vi "Add Value.vi"(8 "error in (no error)":errorcluster, 9 "Value":refnum<class>, 10 "Path":string, 11 "PathTree in":refnum<class "PathTree.lvclass">) -> (0 "error out":errorcluster, 3 "PathTree out":refnum<class "PathTree.lvclass">)   [LabVIEW 2020, in "PathTree.lvlib" / "PathTree.lvclass"]
uses:
  PathTree.lvclass
  PathTreeNode/PathTreeNode.lvclass
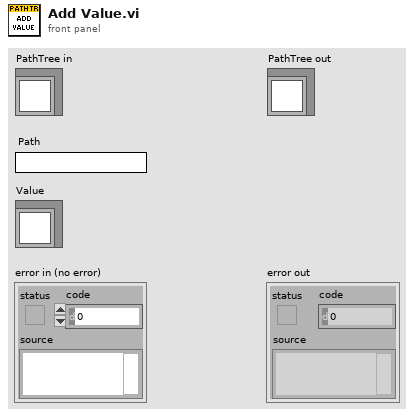
[diagram p1: front panel]
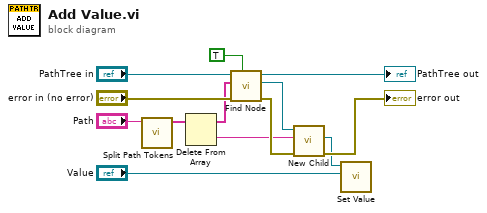
[diagram p0: block diagram]
diagram:
  n1 = call "Split Path Tokens.vi"("Path"="Path") -> ("Tokens"=w11:string[])  [unwired: 10 in]
  n2 = Delete From Array(array=w11) -> (deleted portion=w3:string, array with subset deleted=w5:string[])  [unwired: 2 in]
  n3 = call "Find Node.vi"("Create?"=TRUE, "error in (no error)"="error in (no error)", "Tokens"=w5, "PathTree in"="PathTree in") -> ("error out"=w4:errorcluster, "Node"=w9:refnum<class "PathTreeNode.lvclass">, "PathTree out"=→"PathTree out":refnum<class "PathTree.lvclass">)  [unwired: 5 in]
  n4 = call "New Child.vi"("error in (no error)"=w4, "Child Token"=w3, "PathTreeNode in"=w9) -> ("error out"=→"error out":errorcluster, "Child"=w8:refnum<class "PathTreeNode.lvclass">)  [unwired: 6 in, 1 out]
  n5 = call "Set Value.vi"("Value"="Value", "PathTreeNode in"=w8) -> ()  [unwired: 8 in, 2 out]
